vi "From String Cluster.vi"(0 "Pair":cluster{"Key":string, "Value":string}) -> (2 "Pair":refnum<class "Pair.lvclass">)   [LabVIEW 2018, in "Toolkit.lvlib" / "Data.lvlib" / "Pair.lvclass"]
uses:
  Pair.lvclass
  Pair.lvclass/Pair.ctl
  String/String.lvclass
  D:/Users/cfield/Code/Field R&D Services/Mustache/LabVIEW/trunk/src/Toolkit/Data/Datum/Datum.lvclass
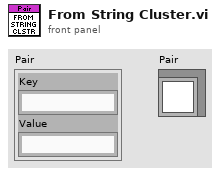
[diagram p1: front panel]
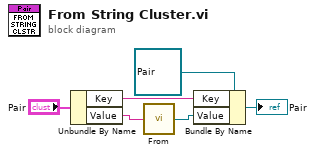
[diagram p0: block diagram]
diagram:
  n1 = Unbundle By Name("Pair") -> ("Key"=w3:string, "Value"=w2:string)
  n2 = call "From.vi"("Value"=w2) -> ("String"=w1:refnum<class "String.lvclass">)
  n3 = Bundle By Name(cluster=refnum<class "Pair.lvclass"> refnum ("Toolkit.lvlib:Data.lvlib:Pair.lvclass"), "Key"=w3, "Value"=w1) -> (→"Pair":refnum<class "Pair.lvclass">)
